vi "Play Frames.vi"(7 "Frames (I:0)":u32[](array[numeric]), 8 "error in (no error)":errorcluster, 10 "Delay per Frame":u32, 11 "Frame Control Ref In":refnum<vi>) -> (0 "error out":errorcluster, 3 "Frame Control Ref Out":refnum<vi>)   [LabVIEW 2018]
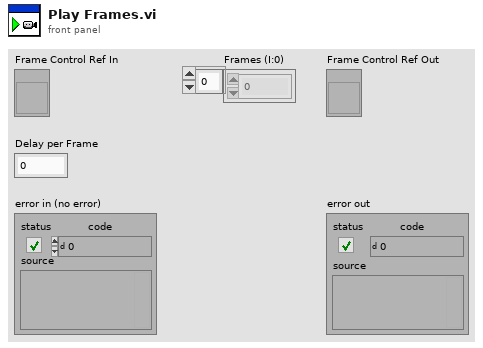
[diagram p1: front panel]
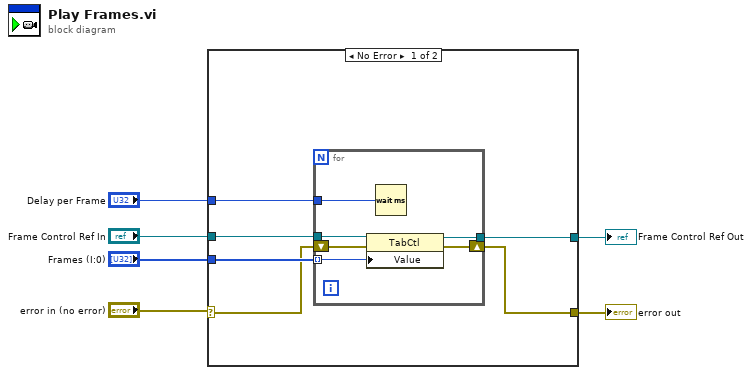
[diagram p0: block diagram]
diagram:
  n1 = case shown="No Error" "error in (no error)" {
    selector: "error in (no error)" -> [w9 w20]
    tunnel: [w8 w20] -> w5
    tunnel: "Frame Control Ref In" -> [w12 w19]
    tunnel: "Frames (I:0)" -> [w11 _]
    tunnel: "Delay per Frame" -> [w10 _]
    tunnel: [w7 w19] -> w1
    frame No Error {
      n2 = for {
        tunnel: w12 -> [w18]
        tunnel: w11 -> [w17] mode=indexing
        tunnel: w10 -> [w16]
        shift-right: [w14] -> w8
        shift-left: w9 -> [w15]
        tunnel: [w13] -> w7
        n3 = property class="TabCtl"(reference=w18, error in=w15, "Value"=w17) -> (reference out=w13:refnum<vi>, error out=w14:errorcluster)
        n4 = Wait (ms)(milliseconds to wait=w16) -> ()  [unwired: 1 out]
      }
    }
    frame Error {
    }
  }
  "error out" <- w5
  "Frame Control Ref Out" <- w1
